vi "PH_SRDG645.destructor.vi"(0 "i ref in":refnum<vi>, 5 "error in":errorcluster) -> (19 "error out":errorcluster)   [LabVIEW 2014, in "PH_SRDG645.lvlib"]
doc: "This is the destructor of a class.\n\nLicense Agreement for this software:\n\nCopyright (C)\nGesellschaft für Schwerionenforschung, GSI\nPlanckstr. 1\n64291 Darmstadt\nGermany\n\nContact: D.Beck@gsi.de \n\nThis program is free software; you can redistribute it and/or modify it under the terms of the \nGNU General Public License as published by the Free Software Foundation; either version 2 of \nthe license, or (at your option) any later version.\n\nThis program is distributed in the hope that it will be useful, but WITHOUT ANY WARRANTY; \nwithout even the implied warranty of MERCHANTABILITY or FITNESS FOR A PARTICULAR PURPOSE. See the GNU General License for more details (http://www.gnu.org).\n\nGesellschaft für Schwerionenforschung, GSI\nPlanckstr. 1, 64291 Darmstadt, Germany\nFor all questions and ideas contact: M.Richter@gsi.de, H.Brand@gsi.de or D.Beck@gsi.de.\nLast update: 16-JUN-2004"
uses:
  PH_SRDG645.lvlib
  CSlibraries-extern/DimLVEvent/LVDimInterface/LVDimInterface.lvlib
  PH_Basics/PH_PSDBWriter/PH_PSDBWriter.lvlib
  PH_Basics/PH_StatusHandler/PH_StatusHandler.lvlib
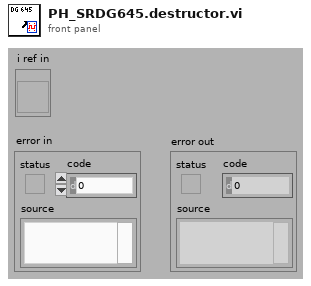
[diagram p1: front panel]
types:
  T1 = typedef "PH_SRDG645.lvlib/PH_SRDG645.i attribute.ctl" = cluster{"GUI Refs":cluster{"Delete":refnum<vi>, "Device Errors":refnum<vi>, "Trigger":refnum<vi>, "Default Name":refnum<vi>, "Firmware Revision":refnum<vi>, "Serial Number":refnum<vi>, "Model":refnum<vi>, "Visa resource name":refnum<vi>}, "Service ID Rate":i32, "Service IDs Channelinfo":i32[], "VISA resource name":refnum<visa-resource-name>, "Device Errors":cluster{"code":i32, "Text":string}[], "Trigger":T2, "Channels":cluster{"T1":T3, "A":T3, "B":T3, "C":T3, "D":T3, "E":T3, "F":T3, "G":T3, "H":T3}, "GUI Refs Channels":refnum<vi>[], "Outputs":cluster{"AB":cluster{"Level Offset [V]":dbl, "Amplitue [V]":dbl, "Polarity":i32}, "CD":cluster{"Level Offset [V]":dbl, "Amplitue [V]":dbl, "Polarity":i32}, "EF":cluster{"Level Offset [V]":dbl, "Amplitue [V]":dbl, "Polarity":i32}, "GH":cluster{"Level Offset [V]":dbl, "Amplitue [V]":dbl, "Polarity":i32}, "T0":cluster{"Level Offset [V]":dbl, "Amplitue [V]":dbl, "Polarity":i32}}, "GUI Refs Outputs":refnum<vi>[], "Serial Number":string, "Firmweare Revision":string, "Model":string}
  T2 = typedef "PH_SRDG645.lvlib/PH_SRDG645.Trigger.ctl" = cluster{"Source":i32, "Rate [Hz]":dbl, "Level [V]":dbl}
  T3 = typedef "PH_SRDG645.lvlib/PH_SRDG645.Channel Settings.ctl" = cluster{"Delay [s]":dbl, "relative to":i32}
  T4 = enum16{"SetAttribute", "GetAttribute", "CreateAttribute", "DestroyAttribute", "DestroyAllAtributes"}
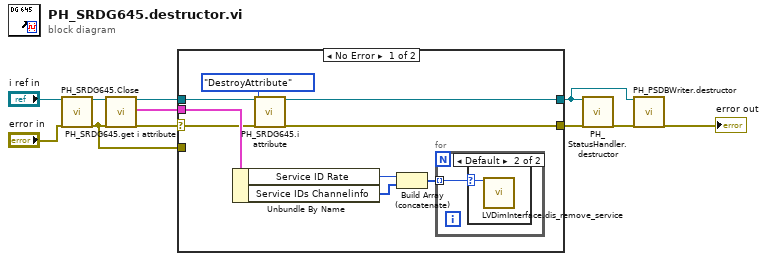
[diagram p0: block diagram]
diagram:
  n1 = call "PH_SRDG645.Close.vi"("i ref in"="i ref in", "error in"="error in") -> ("i ref out"=w7:refnum<vi>, "error out"=w1:errorcluster)  [unwired: 16 in]
  n2 = call "PH_SRDG645.get i attribute.vi"("i ref in"=w7, "error in (no error)"=w1) -> ("i ref out"=w9:refnum<vi>, "i attribute"=w8:T1, "error out"=w2:errorcluster)  [unwired: 15 in]
  n3 = case shown="No Error" w2 {
    selector: w2 -> [w12 _]
    tunnel: [w19 w23] -> w11
    tunnel: w9 -> [w18 w24]
    tunnel: w8 -> [w17 _]
    tunnel: [w13 w24] -> w3
    tunnel: w1 -> [_ w23]
    frame No Error {
      n4 = Unbundle By Name(w17) -> ("Service ID Rate"=w15:i32, "Service IDs Channelinfo"=w14:i32[])
      n5 = call "PH_SRDG645.i attribute.vi"("VI Refnum"=w18, "Action"=T4."DestroyAttribute", "error in (no error)"=w12) -> ("VI Refnum out"=w13:refnum<vi>, "error out"=w19:errorcluster)  [unwired: 14 in, 1 out]
      n6 = Build Array (concatenate)(w15, w14) -> (w16:i32[])
      n7 = for {
        tunnel: w16 -> [w21] mode=indexing
        n8 = case shown="Default" w21 {
          selector: w21 -> [_ w22]
          frame -1 {
          }
          frame Default {
            n9 = call "LVDimInterface.dis_remove_service.vi"("my_serviceID"=w22) -> ()  [unwired: 18 in, 1 out]
          }
        }
      }
    }
    frame Error {
    }
  }
  n10 = call "PH_StatusHandler.destructor.vi"("i ref in"=w3, "error in(no error)"=w11) -> ("error out"=w4:errorcluster)  [unwired: 17 in]
  n11 = call "PH_PSDBWriter.destructor.vi"("i ref in"=w3, "error in(no error)"=w4) -> ("error out"=→"error out":errorcluster)  [unwired: 17 in]
